vi "GraphToImage.vi"() -> ()   [LabVIEW 2012]
panel:
  in  "path to PNG file":path=path "C:/test.png"
  out "Intensity Graph":dbl[][](graph)
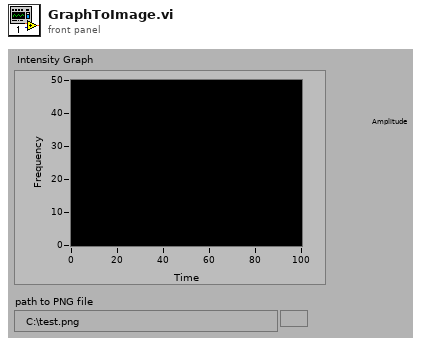
[diagram p1: front panel]
types:
  T1 = typedef "imagedata.ctl" = cluster{"image type":i32, "image depth":i32, "image":u8[], "mask":u8[], "colors":u32[], "Rectangle":cluster{"left":i16, "top":i16, "right":i16, "bottom":i16}}
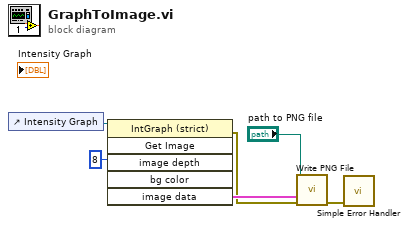
[diagram p0: block diagram]
diagram:
  n1 = control-ref of="Intensity Graph"() -> (w6:refnum<vi>)
  n2 = invoke class="IntGraph (strict)" method="Get Image"(reference=w6, "image depth"=8) -> (error out=w2:errorcluster, "image data"=w4:T1)  [unwired: 4 in, 4 out]
  n3 = call <vilib>:"Write PNG File.vi"("error in (no error)"=w2, "image data"=w4, "path to PNG file"="path to PNG file") -> ("error out"=w1:errorcluster)  [unwired: 7 in, 1 out]
  n4 = call <vilib>:"Simple Error Handler.vi"("error in (no error)"=w1) -> ()  [unwired: 4 in, 5 out]
